vi "Find facing direction.vi"(8 "Desired Task Coordinates (cm)":dbl[](array[numeric]), 11 "Motion History In":dbl[][](array[numeric])) -> (0 "Facing Direction (deg)":dbl, 3 "Motion History Out":dbl[][](array[numeric]))   [LabVIEW 2018]
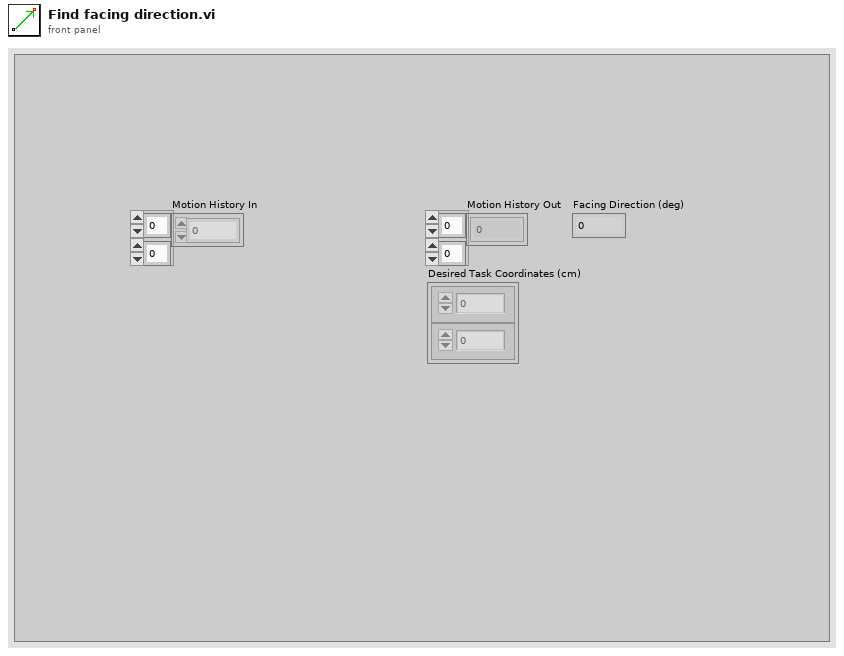
[diagram p1: front panel]
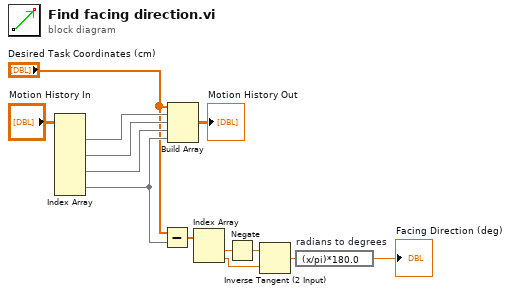
[diagram p0: block diagram]
diagram:
  n1 = Index Array(array="Motion History In") -> (element #1=w7:dbl[], element #2=w8:dbl[], element #3=w9:dbl[], element #4=w6:dbl[])  [unwired: 8 in]
  n2 = Subtract(x="Desired Task Coordinates (cm)", y=w6) -> (x-y=w13:dbl[])
  n3 = Build Array("Desired Task Coordinates (cm)", w7, w8, w9, w6) -> (→"Motion History Out":dbl[][])
  n4 = Index Array(array=w13) -> (element #1=w12:dbl, element #2=w11:dbl)  [unwired: 2 in]
  n5 = Negate(x=w12) -> (-x=w10:dbl)
  n6 = Inverse Tangent (2 Input)(1:w11, 2:w10) -> (0:w5:dbl)
  n7 = expression code="(x/pi)*180.0" "radians to degrees"(w5) -> (→"Facing Direction (deg)":dbl)
